vi "Crc16.vi"(3 "Habilita":bool=TRUE, 5 "tx_rx_buf":string) -> (0 "crc_lo":u8, 1 "crc_hi":u8, 2 "Habilita OUT":bool)   [LabVIEW 2018]
panel:
  out "size(s)":i32
  in  "idx":u8
  out "unsigned byte array":u8[](array[numeric])=[22, 2, 1, 0, 83, 0, 0, 48, 50, 47, 48, 53, 47, 48, 57, 32, 32, 49, 58, 52, 50, 58, 48, 56, 0, 49, 51, 32, 50, 55, 32, 49, 51, 0, 45, 49, 50, 32, 52, 53, 32, 50, 48, 0, 48, 48, 49, 48, 46, 56, 48, 32, 48, 48, 56, 48, 46, 48, 52, 32, 78, 83, 32, 48, 46, 50, 55, 48, 32, 22, 3] format="%x"
  in  "crc16_tab_hi":u8[](array[numeric])=array[5898 elements] format="%x"
  in  "crc16_tab_lo":u8[](array[numeric])=array[6635 elements] format="%x"
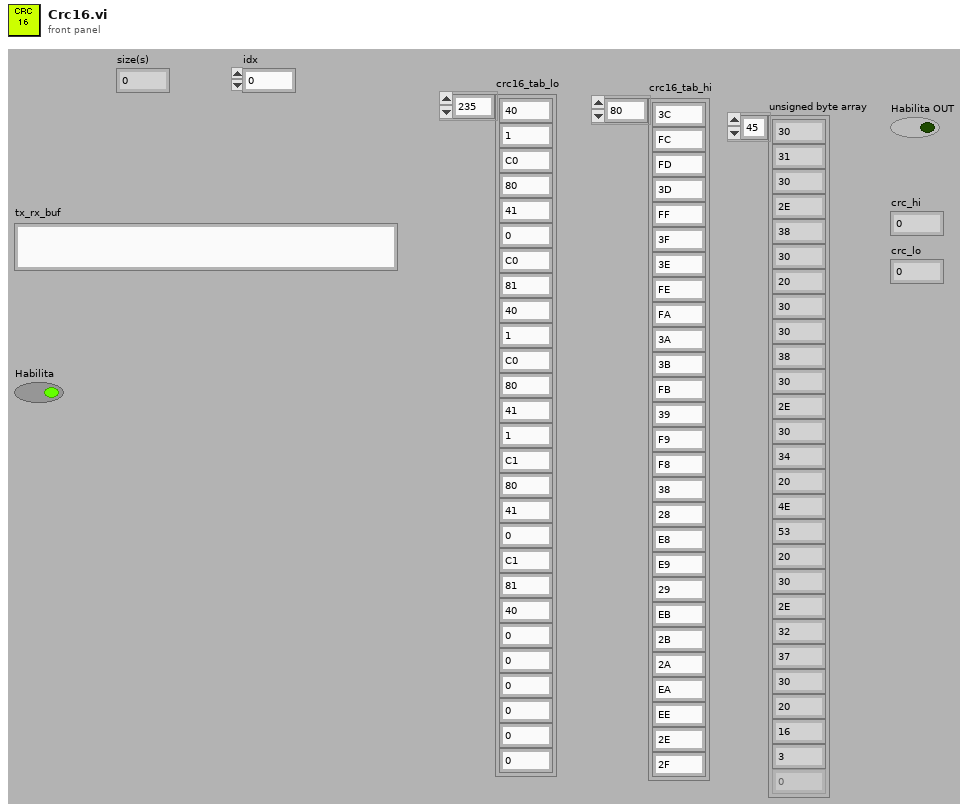
[diagram p1: front panel]
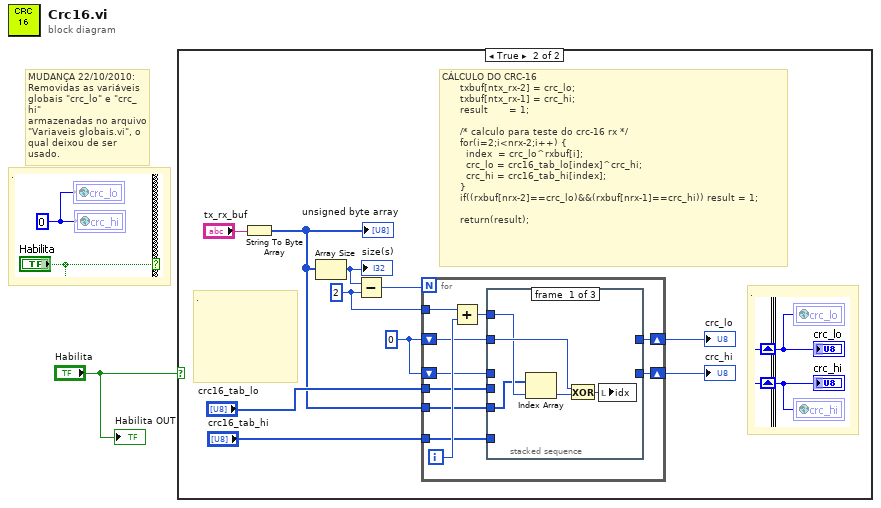
[diagram p0: block diagram]
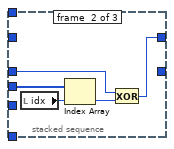
[diagram p3: hidden frame]
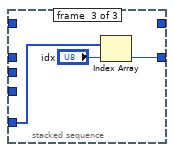
[diagram p4: hidden frame]
diagram:
  # "MUDANÇA 22/10/2010:\nRemovidas as variáveis globais \"crc_lo\" e \"crc_hi\"\narmazenadas no arquivo \"Variaveis globais.vi\", o\nqual deixou de ser usado."
  # "."
  n1 = case shown="True" "Habilita" {
    frame False {
    }
    frame True {
      w2 = 0
      w10 = 2
      # "CÁLCULO DO CRC-16\n      txbuf[ntx_rx-2] = crc_lo;\n      txbuf[ntx_rx-1] = crc_hi;\n      result       = 1;\n\n      /* calculo para teste do crc-16 rx */\n      for(i=2;i<nrx-2;i++) {\n        index  = crc_lo^rxbuf[i];\n        crc_lo = crc16_tab_lo[index]^crc_hi;\n        crc_hi = crc16_tab_hi[index];\n      }\n      if((rxbuf[nrx-2]==crc_lo)&&(rxbuf[nrx-1]==crc_hi)) result = 1;\n\n      return(result);"
      # "."
      # "."
      n2 = String To Byte Array(string="tx_rx_buf") -> (unsigned byte array=w5:u8[])
      "unsigned byte array" <- w5
      n3 = Array Size(array=w5) -> (size(s)=w7:i32)
      "size(s)" <- w7
      n4 = Subtract(x=w7, y=w10) -> (x-y=w11:i32)
      n5 = for {
        N: w11 -> [_]
        shift-right: [w14] -> w4
        shift-left: w2 -> [w19]
        shift-right: [w12] -> w3
        shift-left: w2 -> [w15]
        tunnel: w5 -> [w17]
        tunnel: w10 -> [w20]
        tunnel: "crc16_tab_lo" -> [w16]
        tunnel: "crc16_tab_hi" -> [w13]
        i -> [w21]
        n6 = Add(x=w20, y=w21) -> (x+y=w18:i32)
        n7 = stacked-sequence {
          tunnel: w19 -> [w26 _ _]
          tunnel: w18 -> [w25 _ _]
          tunnel: w17 -> [w24 _ _]
          tunnel: w16 -> [_ w30 _]
          tunnel: w15 -> [_ w28 _]
          tunnel: [_ w27 _] -> w14
          tunnel: w13 -> [_ _ w34]
          tunnel: [_ _ w32] -> w12
          frame #0 {
            n8 = Index Array(array=w24, index=w25) -> (element=w23:u8)
            n9 = Exclusive Or(1:w23, 2:w26) -> (0:w22:i32)
            n10 = local write "idx"(w22) -> ()
          }
          frame #1 {
            n11 = local read "idx"() -> (w31:u8)
            n12 = Index Array(array=w30, index=w31) -> (element=w29:u8)
            n13 = Exclusive Or(1:w29, 2:w28) -> (0:w27:i32)
          }
          frame #2 {
            n14 = Index Array(array=w34, index="idx") -> (element=w32:u8)
          }
        }
      }
      "crc_lo" <- w4
      "crc_hi" <- w3
    }
  }
  "Habilita OUT" <- "Habilita"
